vi "Sauna_DIO.vi"(11 "FPGA VI Reference In":refnum<k20>) -> (2 "Kiuas Toggled":bool, 3 "FPGA VI Reference Out":refnum<k20>)   [LabVIEW 2024]
uses:
  <vilib>/Utility/error.llb/Error Cluster From Error Code.vi
  <vilib>/rvi/errors/niLvFpgaAdjustHostInterfaceError.vi
  <vilib>/rvi/interface/nirviReadWriteControl/nirviReadWriteControl.xnode
  NiFpgaLv.dll
  <vilib>/rvi/interface/Simulation/niFpgaSimulationCallBeginRW.vi
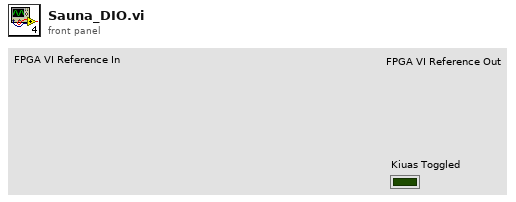
[diagram p1: front panel]
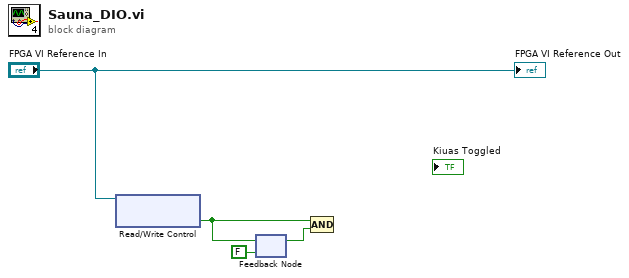
[diagram p0: block diagram]
diagram:
  n1 = xnode "Read/Write Control"("FPGA VI Reference In"="FPGA VI Reference In") -> ("Kiuas Switch"=w3:bool)  [unwired: 1 in, 2 out]
  n2 = feedback-in #1(w3) -> ()
  n3 = feedback #1(FALSE ("Kiuas Switch")) -> (w2:bool)
  n4 = Compound Arithmetic op=AND(w3, w2) -> ()  [unwired: 1 out]
  "FPGA VI Reference Out" <- "FPGA VI Reference In"
